vi "Write to File Week Information ver2.vi"(6 "Actual Per Week":u32, 8 "error in (no error)":errorcluster, 9 "Target Per Week":u32, 10 "Target Cummulative Per Week":u32, 11 "Refnum in":T1) -> (0 "error out":errorcluster, 3 "Refnum out":T1)   [LabVIEW 2018]
uses:
  <vilib>/Utility/config.llb/Config Data RefNum.ctl
  <vilib>/Utility/config.llb/Write Key (U32).vi
  <vilib>/Utility/config.llb/NI_LVConfig.lvlib
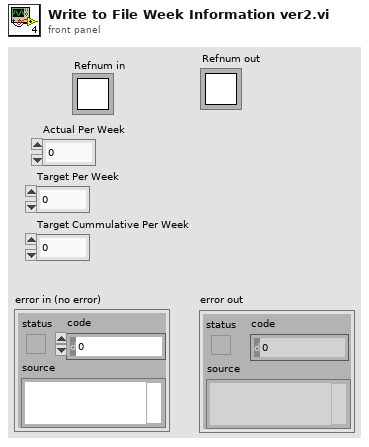
[diagram p1: front panel]
types:
  T1 = typedef "NI_LVConfig.lvlib/Config Data RefNum.ctl" = refnum<k1>
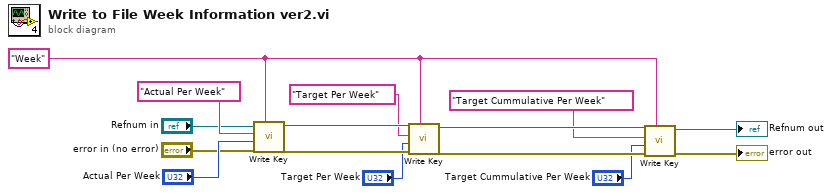
[diagram p0: block diagram]
diagram:
  w11 = "Week" ("section")
  n1 = call-poly <vilib>:"Write Key.vi"("section"=w11, "error in (no error)"="error in (no error)", "value"="Actual Per Week", "key"="Actual Per Week", "refnum"="Refnum in") -> ("error out"=w5:errorcluster, "refnum out"=w10:T1)  [unwired: 4 in, 1 out]
  n2 = call-poly <vilib>:"Write Key.vi"("section"=w11, "error in (no error)"=w5, "value"="Target Per Week", "key"="Target Per Week", "refnum"=w10) -> ("error out"=w6:errorcluster, "refnum out"=w9:T1)  [unwired: 4 in, 1 out]
  n3 = call-poly <vilib>:"Write Key.vi"("section"=w11, "error in (no error)"=w6, "value"="Target Cummulative Per Week", "key"="Target Cummulative Per Week", "refnum"=w9) -> ("error out"=→"error out":errorcluster, "refnum out"=→"Refnum out":T1)  [unwired: 4 in, 1 out]
